vi "MM6.InitDevs.vi"(0 "i ref in":refnum<vi>, 3 "ms timeout (10000)":i32=10000, 5 "error in (no error)":errorcluster) -> (14 "i ref out":refnum<vi>, 17 "timed out":bool, 19 "error out":errorcluster)   [LabVIEW 2014, in "MM6.lvlib"]
doc: "This method should initialize all needed devices. Attention, especially for the scan device is \"Reset\" the first function called."
uses:
  MM6.lvlib
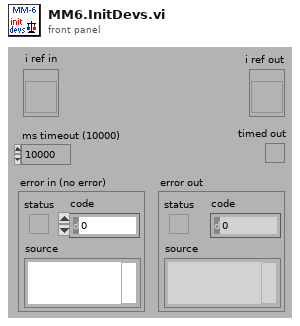
[diagram p1: front panel]
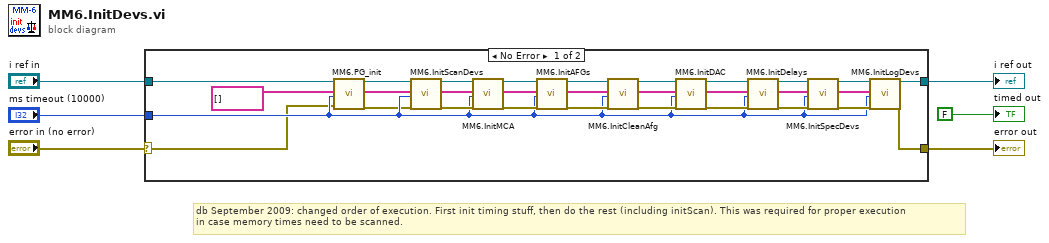
[diagram p0: block diagram]
diagram:
  # "db September 2009: changed order of execution. First init timing stuff, then do the rest (including initScan). This was required for proper execution\nin case memory times need to be scanned."
  n1 = case shown="No Error" "error in (no error)" {
    selector: "error in (no error)" -> [w9 w37]
    tunnel: "i ref in" -> [w15 w38]
    tunnel: [w20 w37] -> w4
    tunnel: [w19 w38] -> w3
    tunnel: "ms timeout (10000)" -> [w11 _]
    frame No Error {
      n2 = call "MM6.PG_init.vi"("i ref in"=w15, "InitObjs"=string[] [], "ms timeout (10000)"=w11, "error in (no error)"=w9) -> ("i ref out"=w14:refnum<vi>, "InitObjs out"=w8:string[], "error out"=w7:errorcluster)  [unwired: 12 in, 1 out]
      n3 = call "MM6.InitScanDevs.vi"("i ref in"=w14, "InitObjs"=w8, "ms timeout (10000)"=w11, "error in (no error)"=w7) -> ("i ref out"=w26:refnum<vi>, "InitObjs out"=w33:string[], "error out"=w34:errorcluster)  [unwired: 12 in, 1 out]
      n4 = call "MM6.InitMCA.vi"("i ref in"=w26, "InitObjs"=w33, "ms timeout (10000)"=w11, "error in (no error)"=w34) -> ("i ref out"=w25:refnum<vi>, "InitObjs out"=w36:string[], "error out"=w35:errorcluster)  [unwired: 12 in, 1 out]
      n5 = call "MM6.InitAFGs.vi"("i ref in"=w25, "InitObjs"=w36, "ms timeout (10000)"=w11, "error in (no error)"=w35) -> ("i ref out"=w24:refnum<vi>, "InitObjs out"=w27:string[], "error out"=w28:errorcluster)  [unwired: 12 in, 1 out]
      n6 = call "MM6.InitCleanAfg.vi"("i ref in"=w24, "InitObjs"=w27, "ms timeout (10000)"=w11, "error in (no error)"=w28) -> ("i ref out"=w23:refnum<vi>, "InitObjs out"=w31:string[], "error out"=w30:errorcluster)  [unwired: 12 in, 1 out]
      n7 = call "MM6.InitDAC.vi"("i ref in"=w23, "InitObjs"=w31, "ms timeout (10000)"=w11, "error in (no error)"=w30) -> ("i ref out"=w22:refnum<vi>, "InitObjs out"=w32:string[], "error out"=w29:errorcluster)  [unwired: 12 in, 1 out]
      n8 = call "MM6.InitDelays.vi"("i ref in"=w22, "InitObjs"=w32, "ms timeout (10000)"=w11, "error in (no error)"=w29) -> ("i ref out"=w13:refnum<vi>, "InitObjs out"=w10:string[], "error out"=w12:errorcluster)  [unwired: 12 in, 1 out]
      n9 = call "MM6.InitSpecDevs.vi"("i ref in"=w13, "InitObjs"=w10, "ms timeout (10000)"=w11, "error in (no error)"=w12) -> ("i ref out"=w18:refnum<vi>, "InitObjs out"=w21:string[], "error out"=w17:errorcluster)  [unwired: 12 in, 1 out]
      n10 = call "MM6.InitLogDevs.vi"("i ref in"=w18, "InitObjs"=w21, "ms timeout (10000)"=w11, "error in (no error)"=w17) -> ("i ref out"=w19:refnum<vi>, "error out"=w20:errorcluster)  [unwired: 12 in, 2 out]
    }
    frame Error {
    }
  }
  "error out" <- w4
  "i ref out" <- w3
  "timed out" <- FALSE ("timed out")
